vi "test Get Interframe Delay.vi"(11 "Test Case In":refnum<class "Test PCANBasic.lvclass">) -> (0 "error out":errorcluster, 3 "Test Case Out":refnum<class "Test PCANBasic.lvclass">)   [LabVIEW 2020, in "Test PCANBasic.lvclass"]
uses:
  Test PCANBasic.lvclass
  Test PCANBasic.lvclass/Test PCANBasic.ctl
  Global PCAN Channel.vi
  source/PCANBasic.lvlib
  Global PCAN Baudrate.vi
  1e10494a-4112-4d37-b82f-f1a7c07c27a4.vi
  source/Set Interframe Delay.vi
  source/Get Interframe Delay.vi
panel:
  out "Interframe Delay":u32 format="%d us"
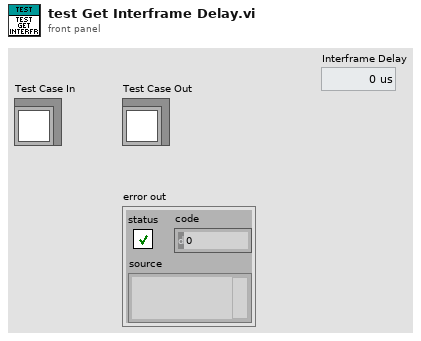
[diagram p1: front panel]
types:
  T1 = typedef "PCANBasic.lvlib/TPCANHandle.ctl" = u16
  T2 = typedef "PCANBasic.lvlib/PCAN Baud.ctl" = u16
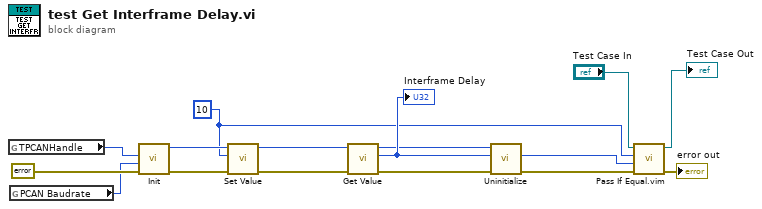
[diagram p0: block diagram]
diagram:
  w1 = u32 10 ("Interframe Delay")
  n1 = global read "Global PCAN Channel.vi" "TPCANHandle"() -> (w9:T1)
  n2 = global read "Global PCAN Baudrate.vi" "PCAN Baudrate"() -> (w8:T2)
  n3 = call "Init.vi"("error in"=errorcluster {"status"=FALSE, "code"=0, "source"=""}, "Baudrate"=w8, "Channel"=w9) -> ("error out"=w10:errorcluster, "TPCANHandle out"=w6:T1)  [unwired: 6 in, 1 out]
  n4 = call-poly "Set Value.vi"("error in"=w10, "Interframe Delay"=w1, "TPCANHandle in"=w6) -> ("error out"=w7:errorcluster, "TPCANHandle out"=w5:T1)  [unwired: 6 in, 1 out]
  n5 = call-poly "Get Value.vi"("error in"=w7, "TPCANHandle in"=w5) -> ("error out"=w11:errorcluster, "Interframe Delay"=w4:u32, "TPCANHandle out"=w2:T1)  [unwired: 6 in, 1 out]
  "Interframe Delay" <- w4
  n6 = call "Uninitialize.vi"("error in"=w11, "TPCANHandle in"=w2) -> ("error out"=w3:errorcluster)  [unwired: 8 in, 1 out]
  n7 = call "Pass If Equal.vim"("error in (no error)"=w3, "Actual"=w4, "Expected"=w1, "LUnit Test Case In"="Test Case In") -> ("error out"=→"error out":errorcluster, "LUnit Test Case Out"=→"Test Case Out":refnum<class "Test PCANBasic.lvclass">)  [unwired: 6 in]
